vi "UDP Server.vi"(8 "error in (no error)":errorcluster, 10 "User Event in":refnum<class "User Event.lvclass">, 11 "UDP Port":u16=5005) -> (0 "error out":errorcluster, 2 "Array":u8[](array[numeric]), 3 "Output":string)   [LabVIEW 2016]
uses:
  User Events/User Event.lvclass
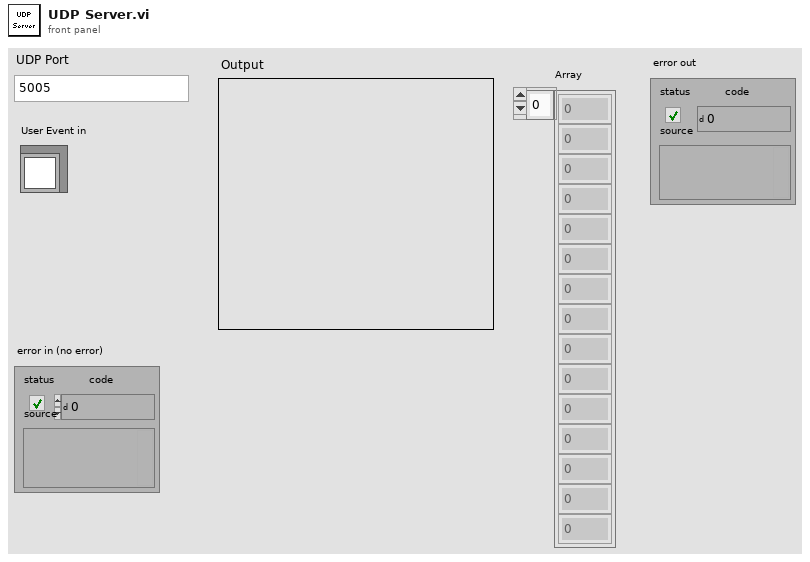
[diagram p1: front panel]
types:
  T1 = typedef "M1M3SupSimUserEvents.ctl" = cluster{"ILCResponse":refnum<user-event>, "StopUDPServer":refnum<user-event>}
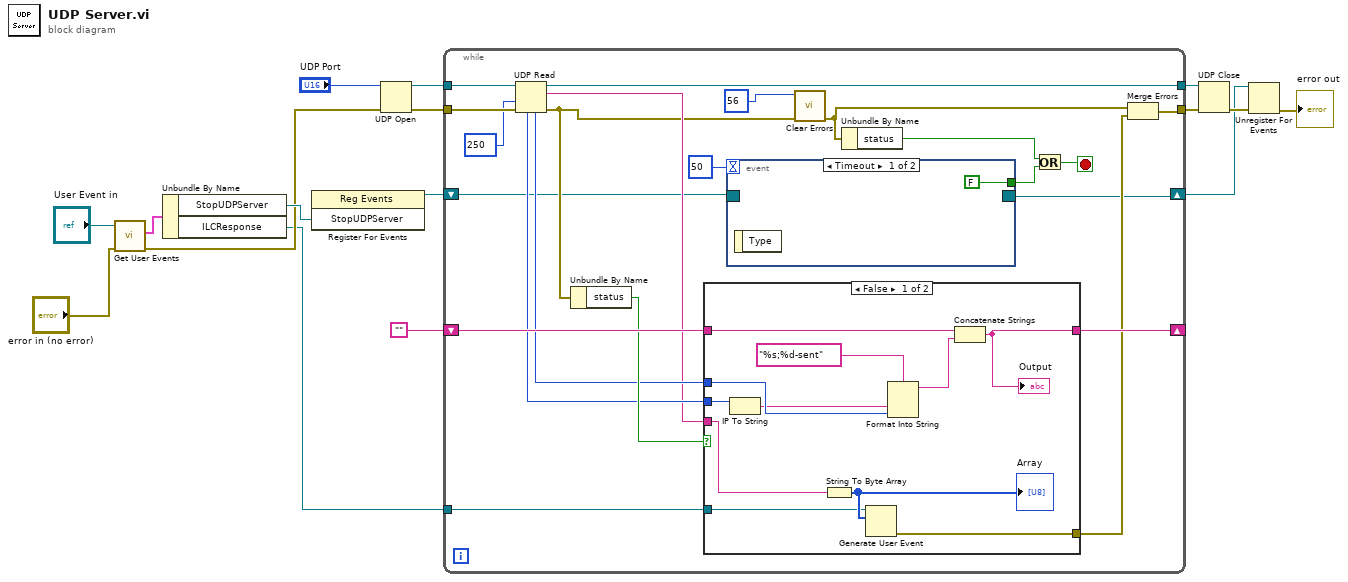
[diagram p0: block diagram]
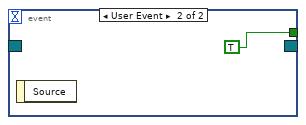
[diagram p2: hidden frame]
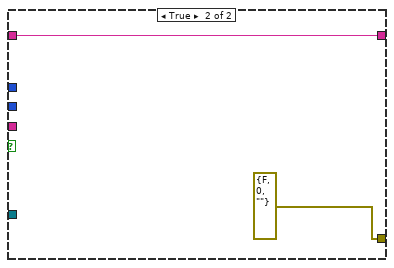
[diagram p3: hidden frame]
diagram:
  n1 = call "Get User Events.vi"("error in (no error)"="error in (no error)", "User Event in"="User Event in") -> ("error out"=w2:errorcluster, "User Events"=w5:T1)  [unwired: 7 in, 1 out]
  n2 = Unbundle By Name(w5) -> ("StopUDPServer"=w4:refnum<user-event>, "ILCResponse"=w1:refnum<user-event>)
  n3 = register-events(w4) -> (reference out=w10:refnum<event-registration>)  [unwired: 2 in, 1 out]
  n4 = UDP Open(8:w2, 11:"UDP Port") -> (port=w15:refnum<k16>, 0:w14:errorcluster)  [unwired: 3 in, 1 out]
  n5 = while {
    tunnel: w15 -> [w38]
    tunnel: w14 -> [w37]
    tunnel: [w23] -> w12
    tunnel: [w35] -> w13
    shift-right: [w33] -> _
    shift-left: "" -> [w34]
    shift-right: [w18] -> w8
    shift-left: w10 -> [w21]
    tunnel: w1 -> [w17]
    stop <- w22 stop-if-true
    n6 = UDP Read(connection ID=w38, timeout ms (25000)=250, 8:w37) -> (data out=w29:string, error out=w28:errorcluster, 3:w35:refnum<k16>, 4:w30:u16, 6:w31:u32)  [unwired: 1 in]
    n7 = Unbundle By Name(w28) -> ("status"=w32:bool)
    n8 = case shown="False" w32 {
      tunnel: w34 -> [w48 w53]
      tunnel: [w46 w53] -> w33
      tunnel: w31 -> [w51 _]
      tunnel: w30 -> [w50 _]
      tunnel: w29 -> [w44 _]
      tunnel: [w41 errorcluster {"status"=FALSE, "code"=0, "source"=""} ("error out")] -> w24
      tunnel: w17 -> [w42 _]
      frame False {
        n9 = IP To String(2:w51) -> (0:w45:string)  [unwired: 1 in]
        n10 = String To Byte Array(string=w44) -> (unsigned byte array=w43:u8[])
        "Array" <- w43
        n11 = Generate User Event(user event=w42, event data cluster=w43) -> (error out=w41:errorcluster)  [unwired: 2 in, 1 out]
        n12 = Format Into String(format string="%s;%d-sent", w45, w50) -> (resulting string=w47:string)  [unwired: 2 in, 1 out]
        n13 = Concatenate Strings(w48, w47) -> (w46:string)
        "Output" <- w46
      }
      frame True {
      }
    }
    n14 = event shown="[0] Timeout" {
      selector: w21 -> [_ _]
      dyn-events: [_ _] -> w18
      timeout: 50 -> [_ _]
      tunnel: [FALSE TRUE] -> w19
      event Timeout {
        n15 = event-data() -> ()  [unwired: 1 in, 1 out]
      }
      event User Event {
        n16 = event-data() -> ()  [unwired: 1 in, 1 out]
      }
    }
    n17 = call <vilib>:"Clear Errors.vi"("error in (no error)"=w28, "specific error code to clear (0: all)"=56) -> ("error out"=w25:errorcluster)  [unwired: 4 in, 1 out]
    n18 = Unbundle By Name(w25) -> ("status"=w26:bool)
    n19 = Or(x=w26, y=w19) -> (x .or. y?=w22:bool)
    n20 = Merge Errors(w25, w24) -> (w23:errorcluster)
  }
  n21 = UDP Close(connection ID=w13, 8:w12) -> (error out=w9:errorcluster)  [unwired: 1 out]
  n22 = Unregister For Events(event registration refnum=w8, error in=w9) -> (error out=→"error out":errorcluster)
